vi "getGeneralLocation.vi"(8 "error in (no error)":errorcluster, 11 "StationKeeping in":refnum<class "StationKeeping.lvclass">) -> (0 "error out":errorcluster, 2 "General Location":T1 {"North" format="%#_10f"; "East" format="%#_8f"}, 3 "StationKeeping out":refnum<class "StationKeeping.lvclass">)   [LabVIEW 2011, in "StationKeeping.lvclass"]
uses:
  StationKeeping.lvclass
  2 Typedefs/UTM Location.ctl
  StationKeeping.lvclass/StationKeeping.ctl
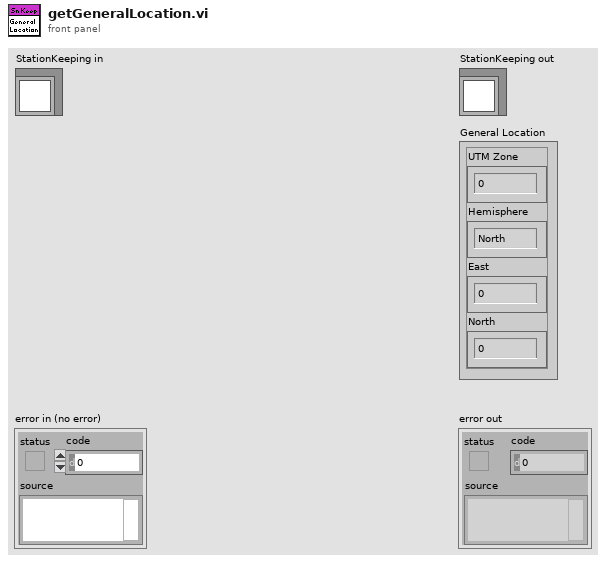
[diagram p1: front panel]
types:
  T1 = typedef "UTM Location.ctl" = cluster{"UTM Zone":dbl, "Hemisphere":enum16{"North", "South"}, "East":dbl, "North":dbl}
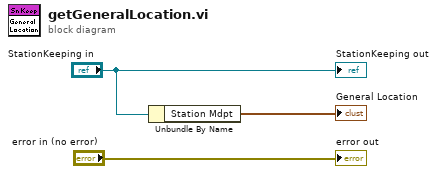
[diagram p0: block diagram]
diagram:
  n1 = Unbundle By Name("StationKeeping in") -> ("Station Mdpt"=→"General Location":T1)
  "error out" <- "error in (no error)"
  "StationKeeping out" <- "StationKeeping in"
